vi "Pre-Build Action.vi"(6 "Top Level/Always Included VIs":path[](array[path]), 7 "Main Destination Path":path, 9 "Target Name":string, 10 "Build Specification Name":string, 11 "Project Path":path) -> (0 "error out":errorcluster)   [LabVIEW 2015]
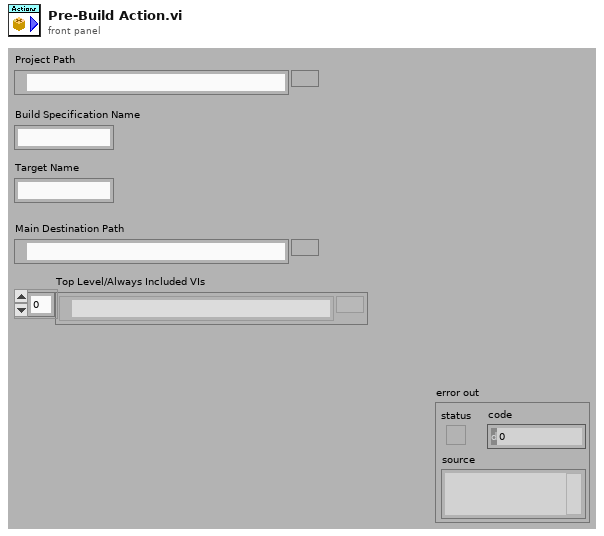
[diagram p1: front panel]
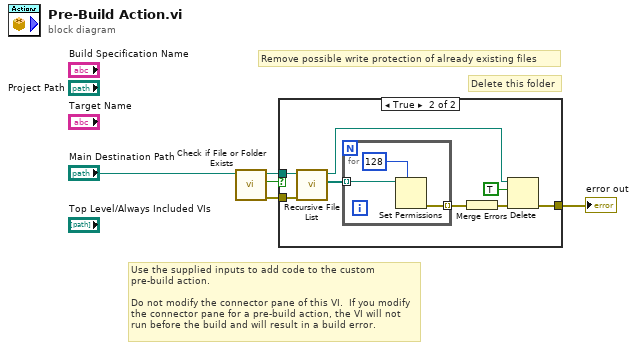
[diagram p0: block diagram]
diagram:
  # "Remove possible write protection of already existing files"
  # "Delete this folder"
  # "Use the supplied inputs to add code to the custom pre-build action.\n\nDo not modify the connector pane of this VI.  If you modify the connector pane for a pre-build action, the VI will not run before the build and will result in a build error."
  n1 = call <vilib>:"Check if File or Folder Exists.vi"("path"="Main Destination Path") -> ("error out"=w4:errorcluster, "file or folder exists?"=w5:bool, "dup path"=w3:path)  [unwired: 8 in]
  n2 = case shown="True" w5 {
    tunnel: w3 -> [_ w10]
    tunnel: w4 -> [w6 w9]
    tunnel: [w6 w13] -> w1
    frame False {
    }
    frame True {
      n3 = call <vilib>:"Recursive File List.vi"("error in (no error)"=w9, "Folder Path"=w10) -> ("All Files in Dir"=w11:path[], "dup Folder Path"=w8:path)  [unwired: 5 in, 3 out]
      n4 = for {
        tunnel: w11 -> [w17] mode=indexing
        tunnel: [w15] -> w12 mode=indexing
        n5 = Set Permissions(7:i16 128 ("permissions"), 11:w17) -> (0:w15:errorcluster)  [unwired: 3 in, 1 out]
      }
      n6 = Merge Errors(w12) -> (w7:errorcluster)
      n7 = Delete(path (use dialog)=w8, entire hierarchy (F)=TRUE, error in=w7) -> (error out=w13:errorcluster)  [unwired: 2 in, 2 out]
    }
  }
  "error out" <- w1
